vi "Moving Average.vi"() -> ()   [LabVIEW 2019]
panel:
  in  "Sensor":dbl(slide) min=-1.0 max=1.0 scale=-1.0..1.0
  out "Plot":cluster{dbl, dbl}(graph)
  in  "Stop":bool
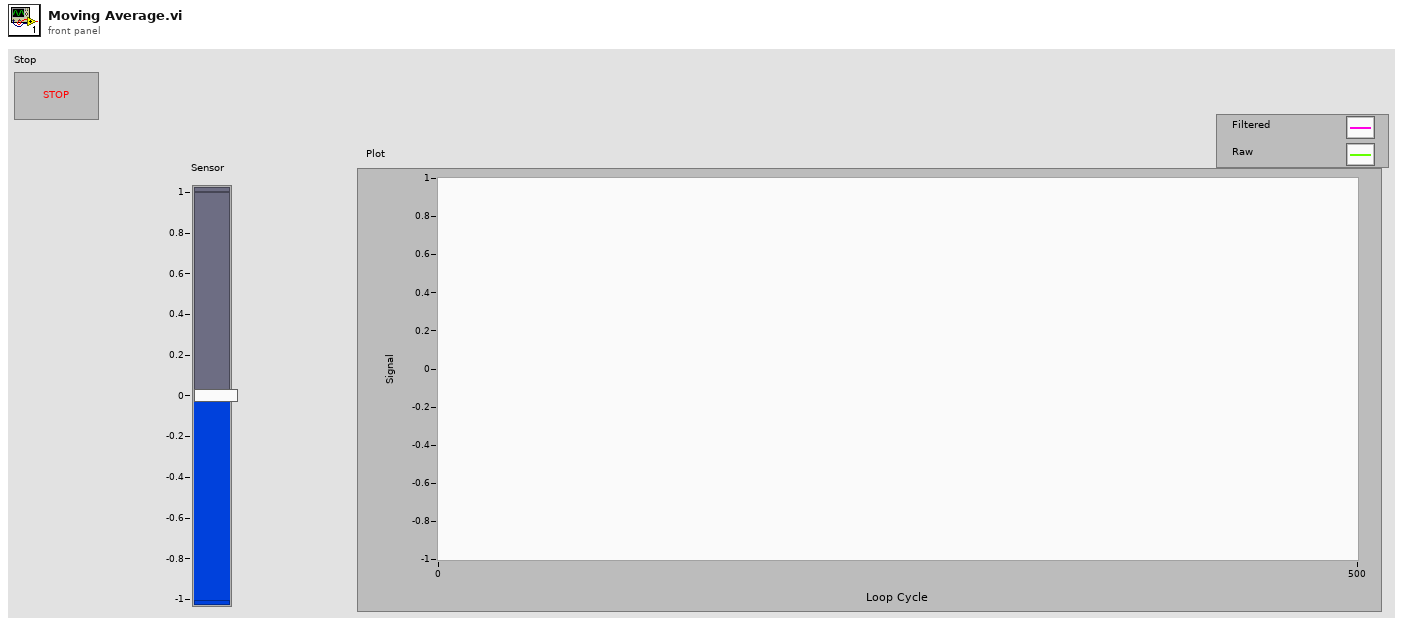
[diagram p1: front panel]
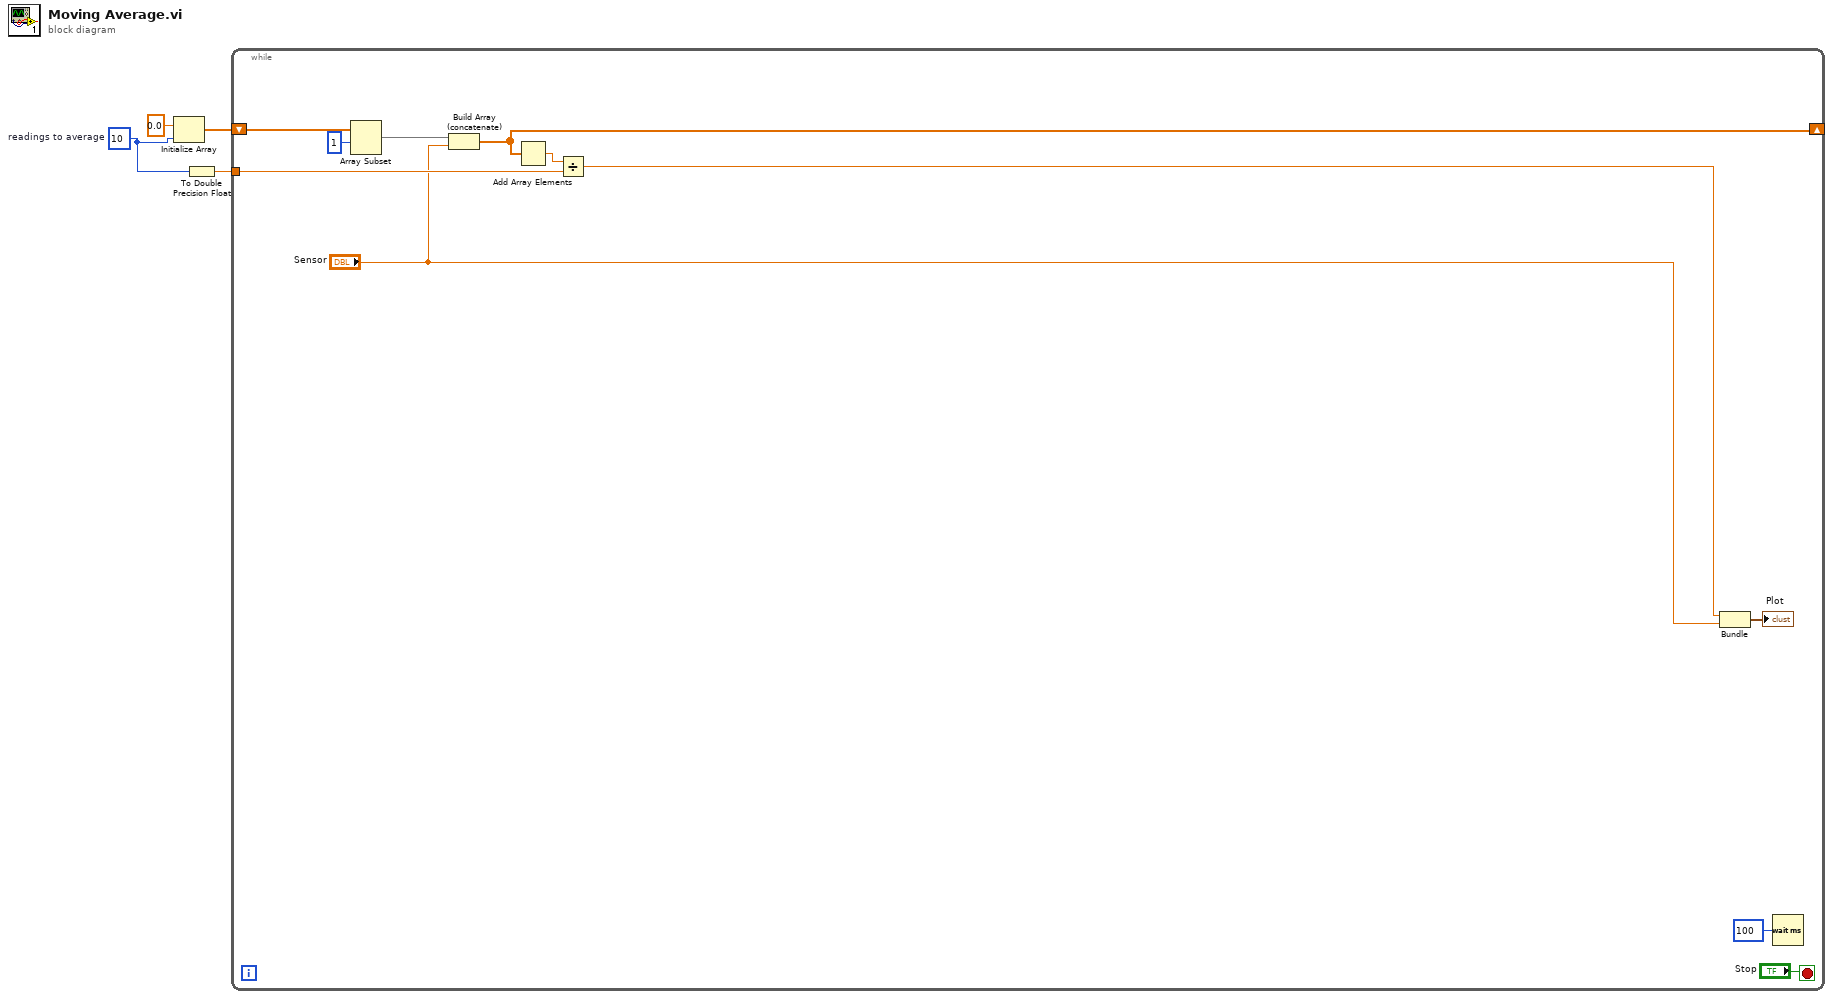
[diagram p0: block diagram]
diagram:
  w2 = 10  # readings to average
  n1 = Initialize Array(0.0 ("element"), w2) -> (w3:dbl[])
  n2 = To Double Precision Float(number=w2) -> (double precision float=w1:dbl)
  n3 = while {
    tunnel: w1 -> [w8]
    shift-right: [w7] -> _
    shift-left: w3 -> [w12]
    stop <- "Stop" stop-if-true
    n4 = Array Subset(array=w12, index=1) -> (w10:dbl[])  [unwired: 1 in]
    n5 = Build Array (concatenate)(w10, "Sensor") -> (w7:dbl[])
    n6 = Add Array Elements(numeric array=w7) -> (sum=w9:dbl)
    n7 = Divide(x=w9, y=w8) -> (x/y=w6:dbl)
    n8 = Bundle(w6, "Sensor"="Sensor") -> (→"Plot":cluster{dbl, "Sensor":dbl})  [unwired: 1 in]
    n9 = Wait (ms)(milliseconds to wait=u32 100) -> ()  [unwired: 1 out]
  }
